vi "OverlayVelocity.vi"(8 "output cluster":T1, 9 "Velocity Out":dbl[](array[numeric]), 10 "Mag Dop Spec":sgl[][](array[numeric])) -> (3 "Array":sgl[][](array[numeric]))   [LabVIEW 2022 SP3]
panel:
  in  "max doppler\nV cm/s":dbl
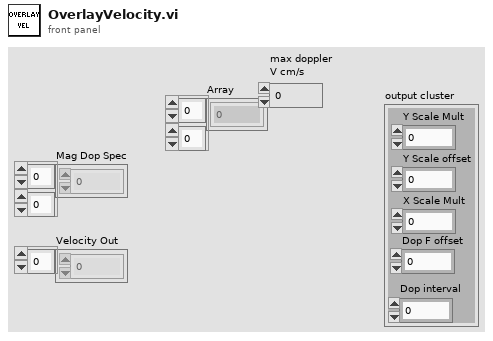
[diagram p1: front panel]
types:
  T1 = cluster{"Y Scale Mult":dbl, "Y Scale offset":dbl, "X Scale Mult":dbl, "Dop F offset":dbl, "Dop interval":dbl}
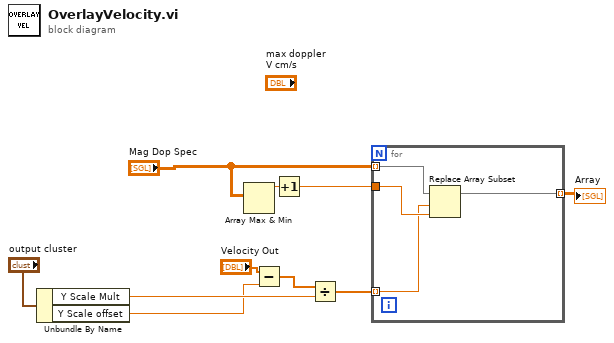
[diagram p0: block diagram]
diagram:
  n1 = Unbundle By Name("output cluster") -> ("Y Scale Mult"=w7:dbl, "Y Scale offset"=w5:dbl)
  n2 = Array Max & Min(array="Mag Dop Spec") -> (max value=w10:sgl)  [unwired: 3 out]
  n3 = Subtract(x="Velocity Out", y=w5) -> (x-y=w8:dbl[])
  n4 = Increment(x=w10) -> (x+1=w3:sgl)
  n5 = Divide(x=w8, y=w7) -> (x/y=w6:dbl[])
  n6 = for {
    tunnel: w3 -> [w14]
    tunnel: [w13] -> w1 mode=indexing
    tunnel: w6 -> [w12] mode=indexing
    tunnel: "Mag Dop Spec" -> [w11] mode=indexing
    n7 = Replace Array Subset(array=w11, new element=w14, index=w12) -> (w13:sgl[])
  }
  "Array" <- w1
